vi "SetSimulatedFreq.vi"(8 "error in (no error)":errorcluster, 9 "Phase offset (deg)":dbl, 10 "Fequency [MHz]":dbl format="%#_8g", 11 "ScopeBase In":refnum<class "ScopeBase.lvclass">) -> (0 "error out":errorcluster, 3 "ScopeBase Out":refnum<class "ScopeBase.lvclass">)   [LabVIEW 2025, in "ScopeBase.lvclass"]
uses:
  ScopeBase.lvclass
  ScopeBase.lvclass/ScopeBase.ctl
  <vilib>/Utility/error.llb/Error Cluster From Error Code.vi
  <vilib>/rvi/errors/niLvFpgaAdjustHostInterfaceError.vi
  <vilib>/rvi/interface/nirviReadWriteControl/nirviReadWriteControl.xnode
  FpgaRef/FpgaRefBase/Common FPGA ref.ctl
  FpgaRef/FpgaRefBase/FpgaRefBase.lvclass
  NiFpgaLv.dll
  <vilib>/rvi/interface/Simulation/niFpgaSimulationCallBeginRW.vi
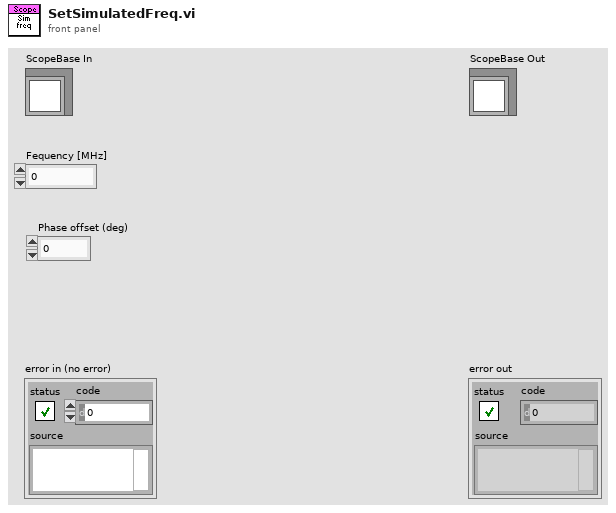
[diagram p1: front panel]
types:
  T1 = typedef "Common FPGA ref.ctl" = refnum<k20>
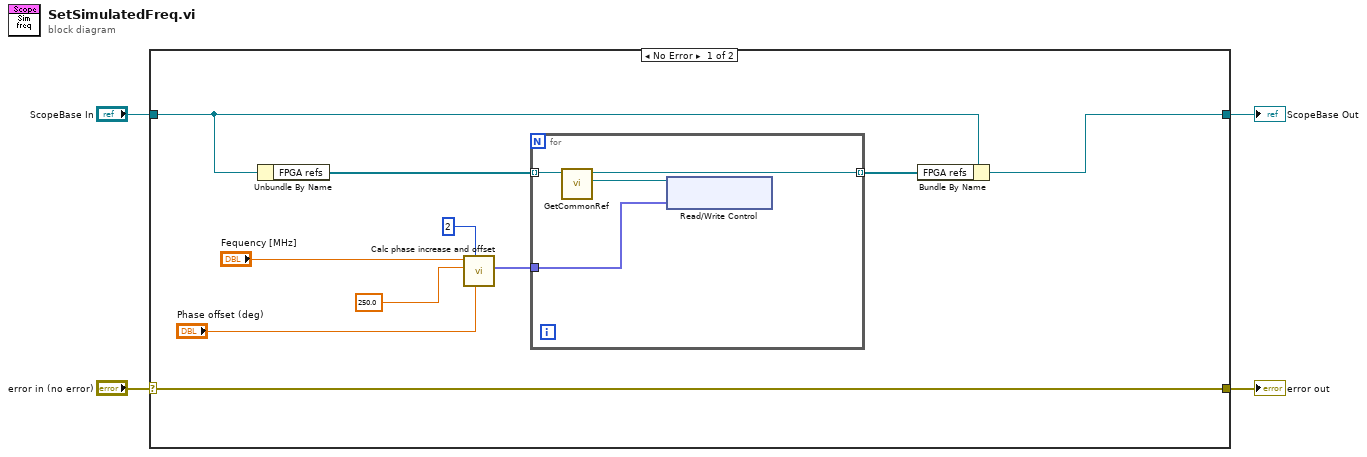
[diagram p0: block diagram]
diagram:
  n1 = case shown="No Error" "error in (no error)" {
    selector: "error in (no error)" -> [w14 w20]
    tunnel: [w14 w20] -> w2
    tunnel: [w5 w19] -> w3
    tunnel: "ScopeBase In" -> [w6 w19]
    frame No Error {
      n2 = Unbundle By Name(w6) -> ("FPGA refs"=w8:refnum<class "FpgaRefBase.lvclass">[])
      n3 = call "Calc phase increase and offset.vi"("Phase offset (deg)"="Phase offset (deg)", "# of DDS"=2, "fclk (MHz)"=250.0 ("fclk (800MHz)"), "f_generated (MHz)"="Fequency [MHz]") -> ("Phase out"=w9:fxp<+,64,64>[])  [unwired: 5 in, 2 out]
      n4 = for {
        tunnel: w9 -> [w18]
        tunnel: w8 -> [w17] mode=indexing
        tunnel: [w15] -> w7 mode=indexing
        n5 = call-dynamic "GetCommonRef.vi"("FpgaRefBase in"=w17) -> ("Common ref"=w16:T1, "FpgaRefBase out"=w15:refnum<class "FpgaRefBase.lvclass">)  [unwired: 8 in, 1 out]
        n6 = xnode "Read/Write Control"("FPGA VI Reference In"=w16, "Simulated phase"=w18) -> ()  [unwired: 1 in, 2 out]
      }
      n7 = Bundle By Name(cluster=w6, "FPGA refs"=w7) -> (w5:refnum<class "ScopeBase.lvclass">)
    }
    frame Error {
    }
  }
  "error out" <- w2
  "ScopeBase Out" <- w3
